vi "Dashboard Main.vi"() -> ()   [LabVIEW 2014]
uses:
  <vilib>/Rock Robotics/WPI/Camera/WPI_CameraSettings Read MJPG.ctl
  <vilib>/Rock Robotics/WPI/Camera/WPI_CameraImageSize.ctl
  Custom VIs/Examples/2015 Vision Example/Vision Support Code/Camera Types.ctl
  <vilib>/event_ctls.llb/eventvkey.ctl
  <vilib>/Rock Robotics/WPI/Dashboard/WPI_DashboardLogging Global.vi
  <vilib>/Rock Robotics/Network Tables/SD Write Number.vi
  <vilib>/Utility/config.llb/Write Key (String).vi
  <vilib>/Utility/config.llb/Write Key (I32).vi
  <vilib>/Utility/config.llb/NI_LVConfig.lvlib
  <vilib>/vision/NI_Vision_Development_Module.lvlib
panel:
  in  "Camera Address 2":string="USB 1"
  in  "Camera Settings 3":T1={"fps"=20, "compression"=30, "Image Size"=enum."320x240"}
  in  "TCP":refnum<k5>
  in  "Rec Mode":enum32{"Stop", "Record", "Playback"}(radio)
  in  "Vision":u16(ring) items=["Camera Off", "USB Camera SW", "USB Camera HW", "IP Camera"]
  out "Camera IP":string
  out "Image Message":string="Timeout in Camera Communications"
  in  "Dashboard Tab":T3(tab)
  in  "Camera Settings":T4={"Frame Rate"=30, "Compression"=30, "Size"=1} {"Frame Rate" scale=1.0..30.0; "Size" items=["640x480", "320x240", "160x120"]}
  out "MotorChart R":cluster{"Numeric":dbl, "Numeric":dbl}(graph)
  out "MotorChart L":T5(graph)
  out "MotorSliders R":cluster{"MotorSlide1":dbl, "MotorSlide2":dbl} {"MotorSlide2" scale=-1.0..1.0 scale format="%#_2e"; "MotorSlide1" scale=-1.0..1.0 scale format="%#_2e"}
  out "MotorSliders L":T6 {"MotorSlide4 2" scale=0.0..14.0 scale format="%#_2e"; "MotorSlide2" scale=-1.0..1.0 scale format="%#_2e"; "MotorSlide1" scale=-1.0..1.0 scale format="%#_2e"}
  out "JS1 Z":dbl(slide) scale=-1.0..1.0 scale format="%#_2e"
  out "JS1 Graph":cluster{"X":dbl, "Y":dbl}[](graph)
  out "JS1 Buttons":T7
  out "JS2 Z":dbl(slide) scale=-1.0..1.0 scale format="%#_2e"
  out "JS2 Graph":cluster{"X":dbl, "Y":dbl}[](graph)
  out "JS2 Buttons":T7
  out "Mode":T8(ring)=enum."Auto Disabled"
  in  "DB Camera Config":bool
  out "fps":dbl format="%#.1g"
  out "Mbps":dbl format="%#.1g"
  out "Mbps 2":bool
  in  "Carpet Color":T9(tab)
  in  "Red":T10={"Hue"={231.0, 14.0}, "Sat"={83.0, 255.0}, "Val"={52.5, 255.0}} {"Hue" scale=0.0..255.0 scale format="%#_3g"}
  in  "Blue":T10={"Hue"={119.0, 181.0}, "Sat"={33.0, 255.0}, "Val"={48.571428571428584, 255.0}} {"Hue" scale=0.0..255.0 scale format="%#_3g"}
  in  "Camera Type":T11=enum."MS HD3000 square"
  in  "Score Threshold":dbl=75.0
  in  "Annotate":bool=TRUE
  in  "Source":enum32{"Files", "Camera"}(tab)
  in  "Images":i32(listbox)
  in  "Folder Location":path=path "Sample Images/KicoffFilmingVision"
  in  "Camera Settings 2":T1={"fps"=20, "compression"=30, "Image Size"=enum."320x240"}
  in  "Camera Address":string="USB 1"
  in  "Show Mask?":bool
  in  "Limit Tests?":bool=TRUE
  in  "Show Carpet Mask":bool=TRUE
  in  "Aspect Fudge Factor":dbl=1.0
  in  "Tote Color":T10={"Hue"={23.67058792990901, 48.923317529462665}, "Sat"={66.78571428571429, 255.0}, "Val"={48.571428571428584, 255.0}} {"Hue" scale=0.0..255.0 scale format="%#_3g"}
  in  "Image Path":path=path "Sample Images/KicoffFilmingVision"
  in  "image files":string[](array[string])
  out "ms to process":u32
  out "Particles":i32
  out "Detected Totes":T12(array[cluster]) {"Normalized Rect"."Numeric 5" format="%#_2g"; "Normalized Rect"."Numeric 3" format="%#_2g"; "Normalized Rect"."Numeric 2" format="%#_2g"; "Normalized Rect"."Numeric" format="%#_2g"}
  out "Sorted Scores":T13(array[cluster]) {"Carpet" format="%#_3g"; "S" format="%#_3g"; "Trapezoid %" format="%#_3g"; "L" format="%#_3g"; "Area to CH" format="%#_3g"; "X" format="%#_3g"; "Y" format="%#_3g"}
  in  "Precision %":dbl(slide) scale=0.0..100.0
  in  "Test Slider":dbl(slide) scale=0.0..100.0 scale format="%#_3g"
  in  "On/Off":bool caption="Solenoid"
  in  "Test Name":u16(ring) items=["Select the test to run...", "Example Test", "-------------------------------", "List of tests is built in robot code.", "Replace with your own automated tests."]
  in  "Test Tree":string(tree)
  in  "Motor":cluster{"Value":dbl, "Enable":bool} {"Value" scale=-1.0..1.0 scale format="%#_3g"}
  out "Progress":T14 {"Test Progress" scale=0.0..100.0}
  in  "Rev/Fwd":cluster{"Forward":bool, "Reverse":bool}
  in  "Test Ring":u16(ring) items=["Monochrome", "Color"]
  in  "Listbox":i32(listbox)
  out "Tree":string(tree)
  out "Camera Image":T15(plugin-control)
  out "Boolean":bool
  # "Left"
  # "Front"
  # "Right"
  # "Battery"
  # "Aspect Ratio"
  # "Density Profile"
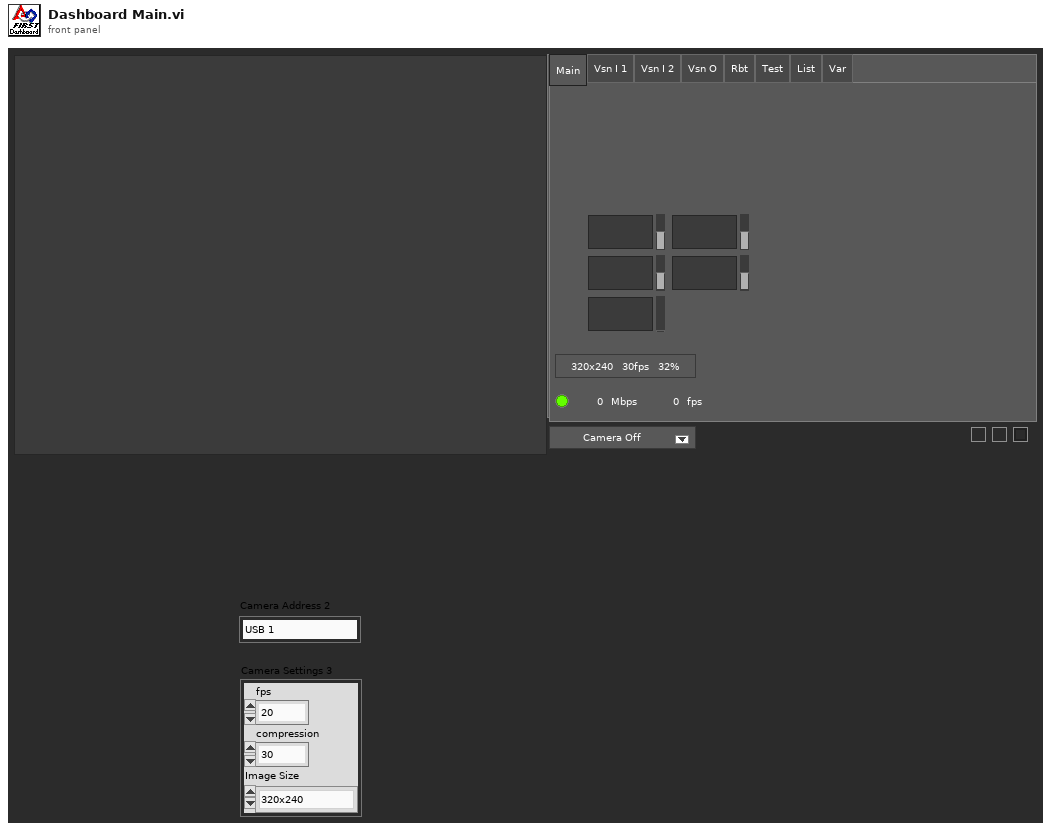
[diagram p1: front panel]
types:
  T1 = typedef "WPI_CameraSettings Read MJPG.ctl" = cluster{"fps":i32, "compression":i32, "Image Size":T2}
  T2 = typedef "WPI_CameraImageSize.ctl" = enum16{"640x480", "320x240", "160x120", "Custom"}
  T3 = enum32{"Main", "Vsn I 1", "Vsn I 2", "Vsn O", "Rbt", "Test", "List", "Var"}
  T4 = cluster{"Frame Rate":i32, "Compression":i32, "Size":u16}
  T5 = cluster{"Numeric":dbl, "Numeric":dbl, "Battery V":dbl}
  T6 = cluster{"MotorSlide1":dbl, "MotorSlide2":dbl, "MotorSlide4 2":dbl}
  T7 = cluster{bool, bool, bool, bool, bool, bool, bool, bool, bool, bool, bool, bool}
  T8 = enum8{"Tele-Op Disabled", "Tele-Op Enabled", "Auto Disabled", "Auto Enabled", "Test Disabled", "Test Enabled", "Disconnected", "No Code", "E-Stop"}
  T9 = enum32{"Red Carpet Color", "Blue Carpet Color", "None"}
  T10 = cluster{"Hue":cluster{dbl, dbl}, "Sat":cluster{dbl, dbl}, "Val":cluster{dbl, dbl}}
  T11 = typedef "Camera Types.ctl" = enum16{"206", "1011", "1013", "MS HD3000 square", "MS HD3000 640x480"}
  T12 = cluster{"Distance (ft)":dbl, "Center":cluster{dbl, dbl}, "Normalized Rect":cluster{"Numeric":dbl, "Numeric 2":dbl, "Numeric 3":dbl, "Numeric 5":dbl}}[]
  T13 = cluster{"Rectangle":cluster{"Numeric":dbl, "Numeric 2":dbl, "Numeric 3":dbl, "Numeric 5":dbl}, "Trapezoid %":dbl, "L":dbl, "S":dbl, "Area to CH":dbl, "X":dbl, "Y":dbl, "Carpet":dbl}[]
  T14 = cluster{"Test Progress":u8, "Test Progress Text":string}
  T15 = typedef "IMAQ Image.ctl" = refnum<image>
  T16 = typedef "Particle Parameters" = i32
  T17 = typedef "Image Type" = u32
  T18 = enum32{"Drive", "Basic", "Custom", "Test", "Checklist", "Variables"}
  T19 = cluster{"Camera Image":refnum<vi>, "Dashboard Tab":refnum<vi>, "Boolean":refnum<vi>, "Vision":refnum<vi>, "Rec Mode":refnum<vi>, "Test Slider":refnum<vi>, "On/Off ":refnum<vi>, "Test Ring":refnum<vi>, "Rev/Fwd":refnum<vi>, "Test Name":refnum<vi>, "Motor":refnum<vi>, "Progress":refnum<vi>, "CheckList":refnum<vi>, "Tree":refnum<vi>, "Test Tree":refnum<vi>}
  T20 = cluster{"Error Strings":string, "Disable Counts":cluster{u16, u16}, "Rail Faults":cluster{u16, u16, u16}, "Robot IP":string, "DB Mode":u8, "Event Info":cluster{"Name":string, "Type":u8, "Number":u16, "Replay":u8}, "Camera Addr":string}
  T21 = cluster{"Storage":cluster{"Disk Free":u64, "RAM Block":u32, "RAM free":u32}, "CPU Utilization":cluster{"CPU % ISR":sgl, "CPU % Time Crit":sgl, "CPU % Timed Str":sgl, "CPU % High":sgl, "CPU % Above":sgl, "CPU % Normal":sgl, "CPU % Low":sgl}, "CAN":cluster{"% Bus Utilization":sgl, "Bus Off Cnt":u32, "TX_FIFO Full Cnt":u32, "Receive Error Cnt":u8, "Transmit Error Cnt":u8}, "HID":cluster{"HID Outputs":u32, "Rumble Low":u16, "Rumble High":u16}[]}
  T22 = cluster{"Status bits":cluster{"Test Mode":bool, "Autonomous":bool, "Enabled":bool, "Code Start":bool, "Brownout":bool, "Reserved 2":bool, "Reserved 3":bool, "E-Stop":bool}, "Code Trace":cluster{"Disabled":bool, "TeleOp":bool, "Auto":bool, "Test":bool}, "Controller Type":enum16{"unknown", "cRIO", "roboRio"}, "Code?":enum16{"unknown", "noCode", "code"}, "Battery V":dbl}
  T23 = cluster{"Control Bits":cluster{"TestMode":bool, "Autonomous":bool, "Enabled":bool, "FMS Present":bool, bool, bool, bool, "E-Stop":bool}, "Team Station ":u8, "Countdown":sgl, "Joystick Values":cluster{"Axes":dbl[], "Buttons":bool[], "POVs":i16[]}[]}
  T24 = cluster{"Axes":dbl[], "Buttons":bool[], "POVs":i16[]}[]
  T25 = cluster{"Axes":dbl[], "Buttons":bool[], "POVs":i16[]}
  T26 = cluster{"Buttons[0]":bool, "Buttons[1]":bool, "Buttons[2]":bool, "Buttons[3]":bool, "Buttons[4]":bool, "Buttons[5]":bool, "Buttons[6]":bool, "Buttons[7]":bool, "Buttons[8]":bool, "Buttons[9]":bool, "Buttons[10]":bool, "Buttons[11]":bool}
  T27 = cluster{"Bounding box":cluster{"left":dbl, "top":dbl, "right":dbl, "bottom":dbl}, "Trapezoid":dbl, "Long Aspect":dbl, "Short Aspect":dbl, "Area to CH":dbl, "X Mask":dbl, "Y Mask":dbl, "Carpet":dbl}[]
  T28 = cluster{"Red":cluster{"Hue":cluster{dbl, dbl}, "Sat":cluster{dbl, dbl}, "Val":cluster{dbl, dbl}}, "Blue":cluster{"Hue":cluster{dbl, dbl}, "Sat":cluster{dbl, dbl}, "Val":cluster{dbl, dbl}}}
  T29 = cluster{cluster{"[0]":dbl, "[1]":dbl, "[2]":dbl, "[3]":dbl}, "Score":dbl, "Long Edge Score":dbl, "Short Edge Score":dbl, dbl, "X Score":dbl, "Y Score":dbl, "Carpet":dbl}[]
  T30 = cluster{"Found Totes[0]":cluster{"Distance (ft)":dbl, "Center":cluster{dbl, dbl}, "Normalized Rect":cluster{"Numeric":dbl, "Numeric 2":dbl, "Numeric 3":dbl, "Numeric 5":dbl}}, "Found Totes[1]":cluster{"Distance (ft)":dbl, "Center":cluster{dbl, dbl}, "Normalized Rect":cluster{"Numeric":dbl, "Numeric 2":dbl, "Numeric 3":dbl, "Numeric 5":dbl}}, "Found Totes[2]":cluster{"Distance (ft)":dbl, "Center":cluster{dbl, dbl}, "Normalized Rect":cluster{"Numeric":dbl, "Numeric 2":dbl, "Numeric 3":dbl, "Numeric 5":dbl}}, "Found Totes[3]":cluster{"Distance (ft)":dbl, "Center":cluster{dbl, dbl}, "Normalized Rect":cluster{"Numeric":dbl, "Numeric 2":dbl, "Numeric 3":dbl, "Numeric 5":dbl}}, "Found Totes[4]":cluster{"Distance (ft)":dbl, "Center":cluster{dbl, dbl}, "Normalized Rect":cluster{"Numeric":dbl, "Numeric 2":dbl, "Numeric 3":dbl, "Numeric 5":dbl}}, "Found Totes[5]":cluster{"Distance (ft)":dbl, "Center":cluster{dbl, dbl}, "Normalized Rect":cluster{"Numeric":dbl, "Numeric 2":dbl, "Numeric 3":dbl, "Numeric 5":dbl}}, "Found Totes[6]":cluster{"Distance (ft)":dbl, "Center":cluster{dbl, dbl}, "Normalized Rect":cluster{"Numeric":dbl, "Numeric 2":dbl, "Numeric 3":dbl, "Numeric 5":dbl}}, "Found Totes[7]":cluster{"Distance (ft)":dbl, "Center":cluster{dbl, dbl}, "Normalized Rect":cluster{"Numeric":dbl, "Numeric 2":dbl, "Numeric 3":dbl, "Numeric 5":dbl}}, "Found Totes[8]":cluster{"Distance (ft)":dbl, "Center":cluster{dbl, dbl}, "Normalized Rect":cluster{"Numeric":dbl, "Numeric 2":dbl, "Numeric 3":dbl, "Numeric 5":dbl}}}
  T31 = typedef "NI_LVConfig.lvlib/Config Data RefNum.ctl" = refnum<k1>
  T32 = cluster{"Operation":enum16{"Update", "Clear"}, "Color Box":u32}[]
  T33 = typedef "eventvkey.ctl" = enum16{"ASCII", "Enter", "Return", "Shift", "Ctrl", "Alt", "Cmd", "Opt", "Caps", "NumLock", "Clear", "Break", "Up", "Down", "Left", "Right", "Insert", "Delete", "Home", "End", "PageUp", "PageDown", "Escape", "Help", "Pause", "ScrollLock", "F1", "F2", "F3", "F4", "F5", "F6", "F7", "F8", "F9", "F10", "F11", "F12", "F13", "F14", "F15", "F16", "F17", "F18", "F19", "F20", "F21", "F22", "F23", "F24", "Play", "VolumeUp", "VolumeDown", "Mute", "Two Byte Char"}
  T34 = cluster{"Image Size":bool, "Image Type":bool, "Pixel Value":bool, "ROI Information":bool, "Zoom Factor":bool}
  T35 = enum8{"Enabled", "Disabled", "Disabled and Grayed Out"}
  T36 = cluster{"Operation":enum16{"Update", "Clear"}, "Color Box":u32}
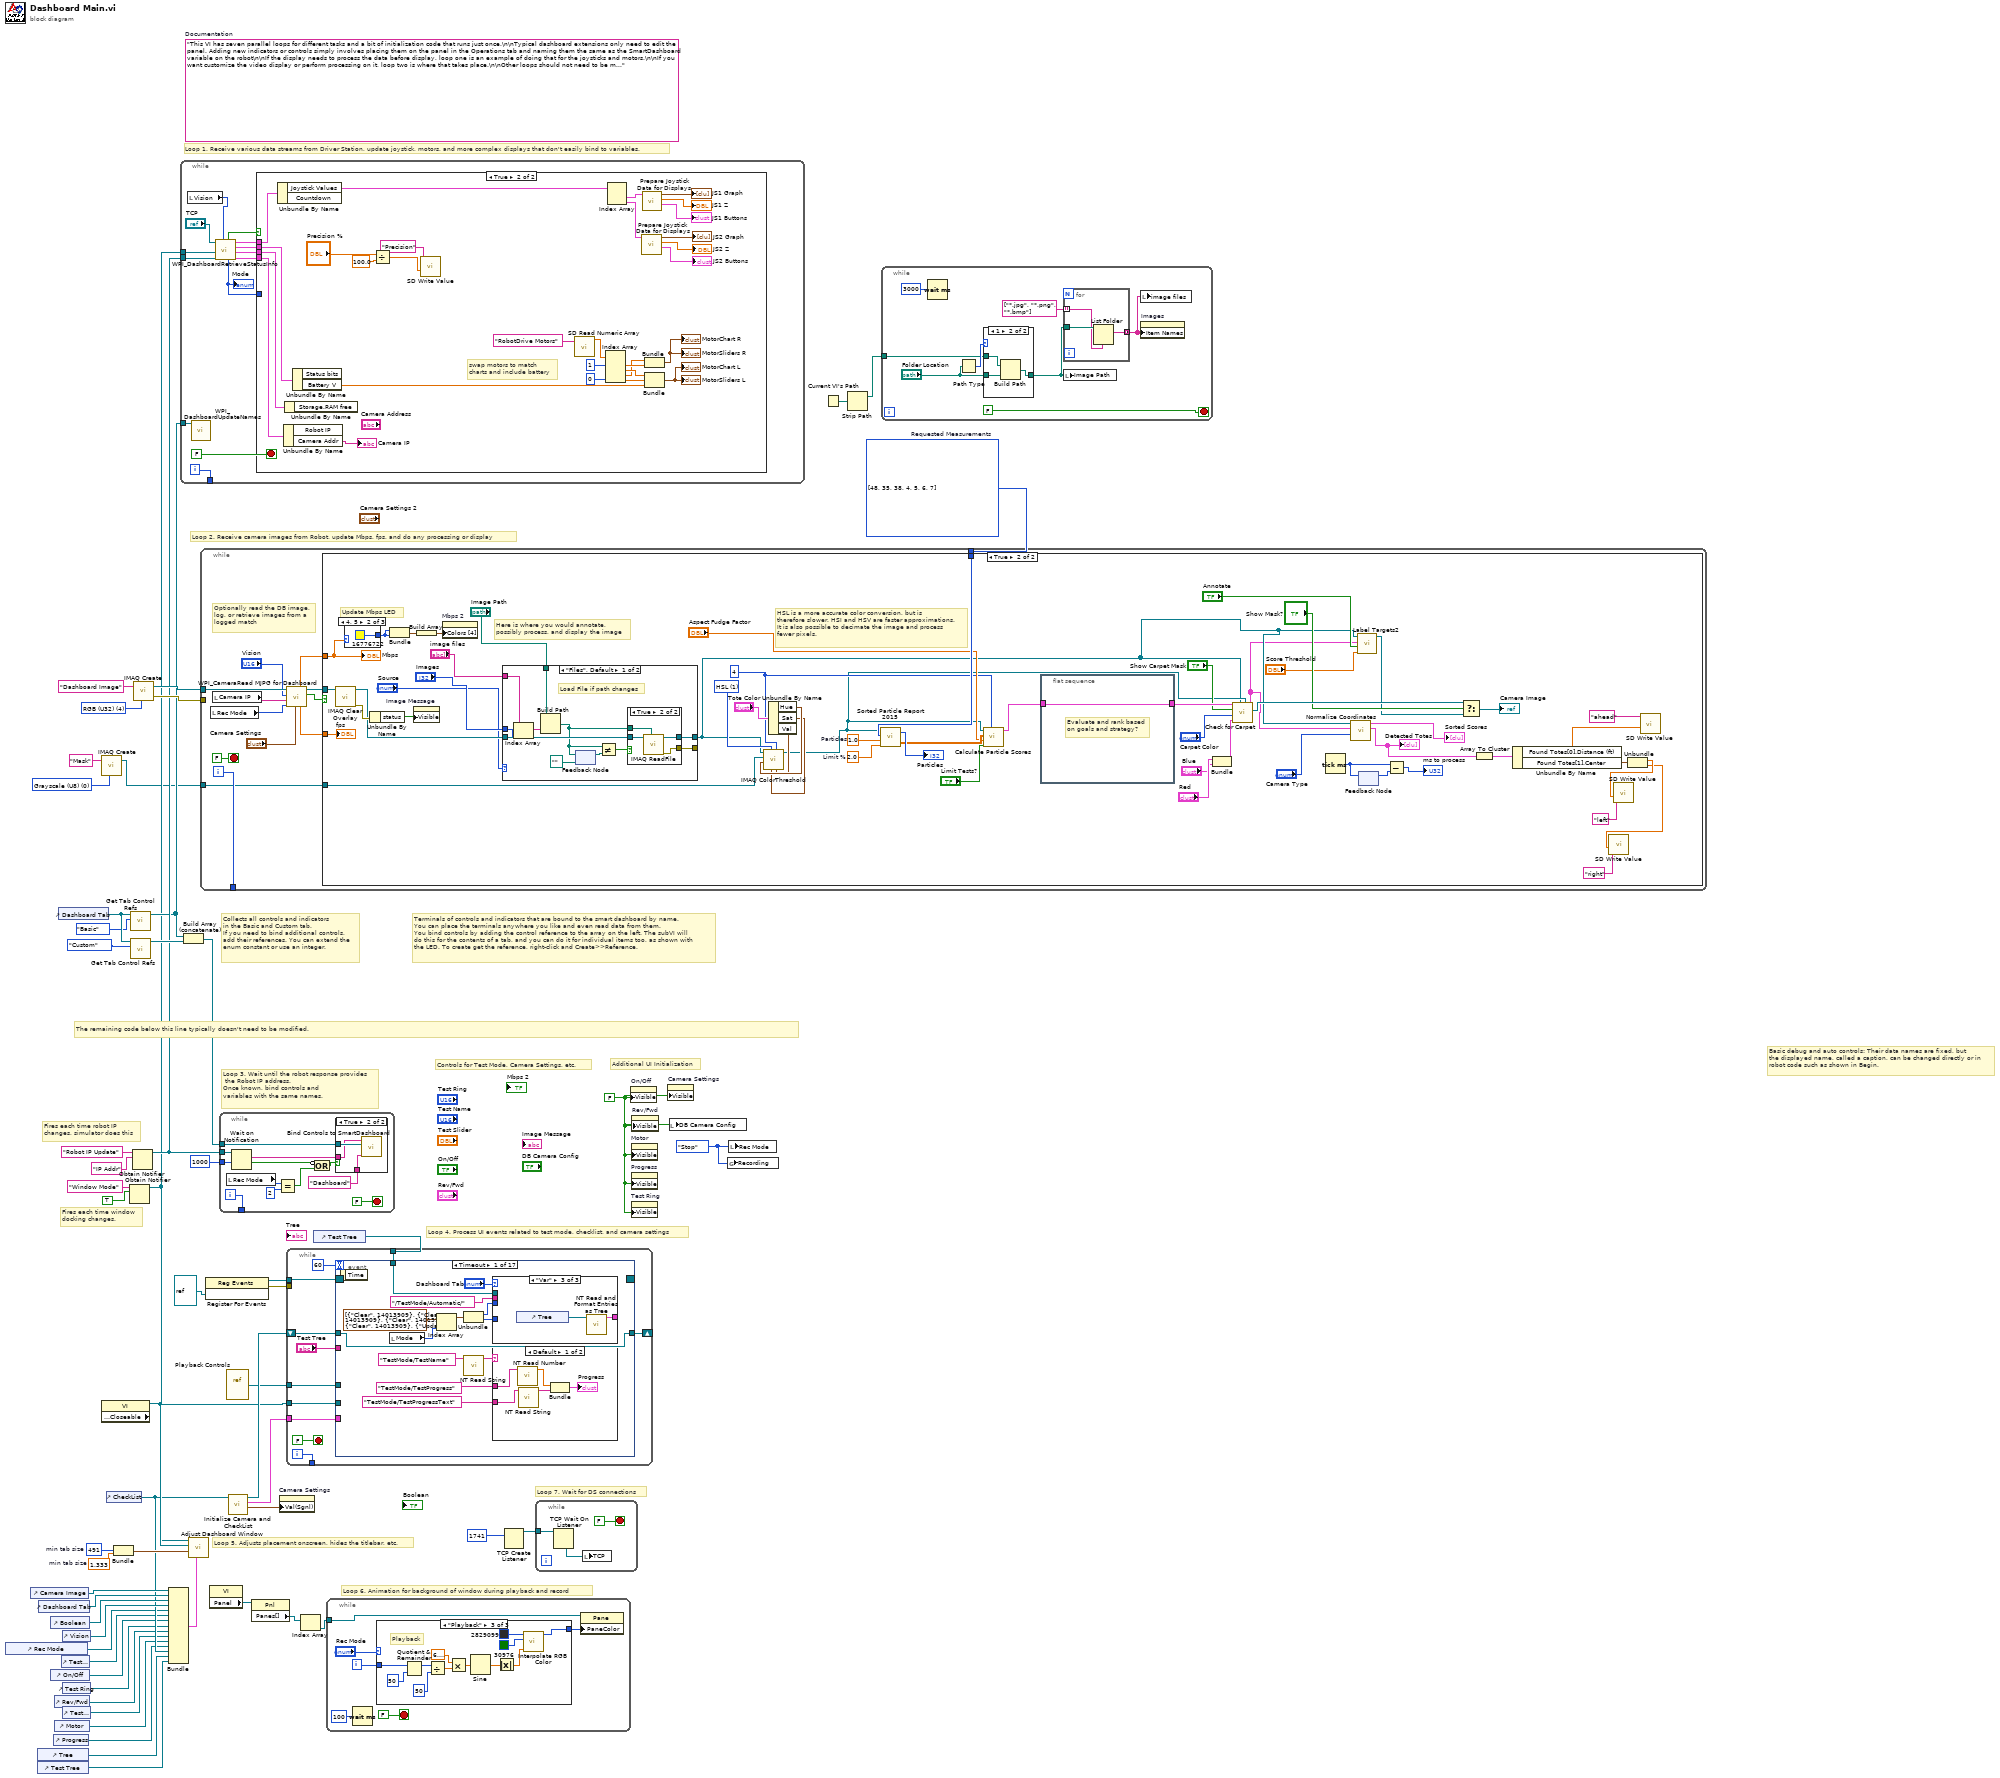
[diagram p0: block diagram]
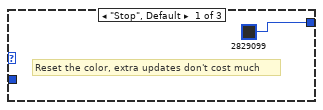
[diagram p4: hidden frame]
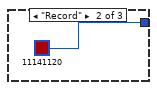
[diagram p5: hidden frame]
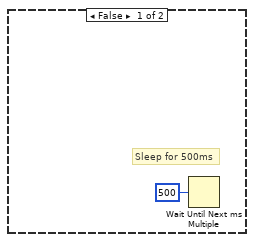
[diagram p7: hidden frame]
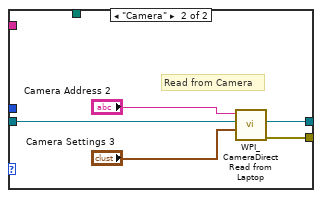
[diagram p9: hidden frame]
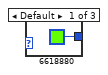
[diagram p10: hidden frame]
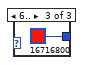
[diagram p11: hidden frame]
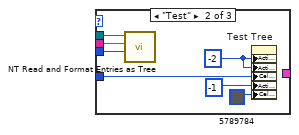
[diagram p13: hidden frame]
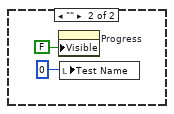
[diagram p14: hidden frame]
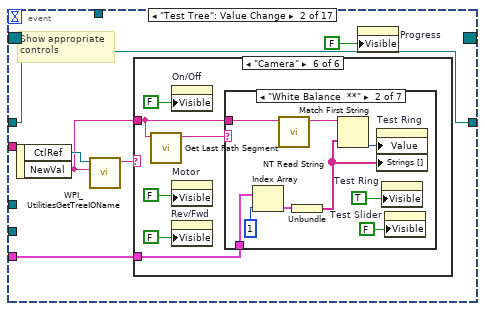
[diagram p15: hidden frame]
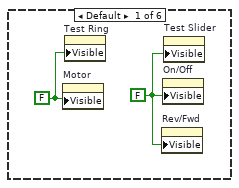
[diagram p16: hidden frame]
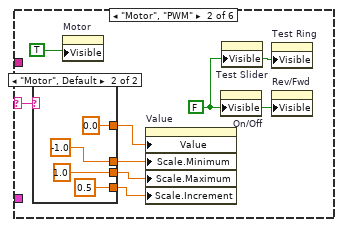
[diagram p17: hidden frame]
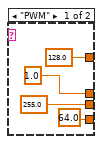
[diagram p18: hidden frame]
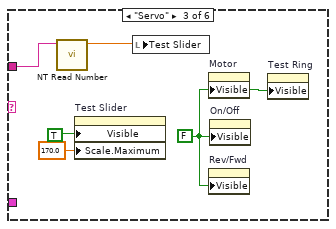
[diagram p19: hidden frame]
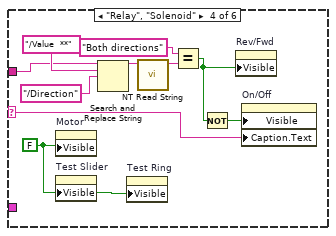
[diagram p20: hidden frame]
diagram:
  w1 = T16[] [48, 35, 38, 4, 5, 6, 7] items=["Center of Mass X", "Center of Mass Y", "First Pixel X", "First Pixel Y", "Bounding Rect Left", "Bounding Rect Top", "Bounding Rect Right", "Bounding Rect Bottom", "Max Feret Diameter Start X", "Max Feret Diameter Start Y", "Max Feret Diameter End X", "Max Feret Diameter End Y", "Max Horiz. Segment Length Left", "Max Horiz. Segment Length Right", "Max Horiz. Segment Length Row", "-", "Bounding Rect Width", "Bounding Rect Height", "Bounding Rect Diagonal", "Perimeter", "Convex Hull Perimeter", "Holes' Perimeter", "Max Feret Diameter", "Equivalent Ellipse Major Axis", "Equivalent Ellipse Minor Axis", "Equivalent Ellipse Minor Axis (Feret)", "Equivalent Rect Long Side", "Equivalent Rect Short Side", "Equivalent Rect Diagonal", "Equivalent Rect Short Side (Feret)", "Average Horiz. Segment Length", "Average Vert. Segment Length", "Hydraulic Radius", "Waddel Disk Diameter", "-", "Area", "Holes' Area", "Particle & Holes' Area", "Convex Hull Area", "Image Area", "-", "Number of Holes", "Number of Horiz. Segments", "Number of Vert. Segments", "-", "Orientation", "Max Feret Diameter Orientation", "-", "% Area/Image Area", "% Area/(Particle & Holes' Area)", "Ratio of Equivalent Ellipse Axes", "Ratio of Equivalent Rect Sides", "-", "Elongation Factor", "Compactness Factor", "Heywood Circularity Factor", "Type Factor", "-", "Sum X", "Sum Y", "Sum XX", "Sum XY", "Sum YY", "Sum XXX", "Sum XXY", "Sum XYY", "Sum YYY", "-", "Moment of Inertia XX", "Moment of Inertia XY", "Moment of Inertia YY", "Moment of Inertia XXX", "Moment of Inertia XXY", "Moment of Inertia XYY", "Moment of Inertia YYY", "Norm. Moment of Inertia XX", "Norm. Moment of Inertia XY", "Norm. Moment of Inertia YY", "Norm. Moment of Inertia XXX", "Norm. Moment of Inertia XXY", "Norm. Moment of Inertia XYY", "Norm. Moment of Inertia YYY", "Hu Moment 1", "Hu Moment 2", "Hu Moment 3", "Hu Moment 4", "Hu Moment 5", "Hu Moment 6", "Hu Moment 7"]  # Requested Measurements
  w4 = T17 0 items=["Grayscale (U8)", "Grayscale (I16)", "Grayscale (SGL)", "Complex (CSG)", "RGB (U32)", "HSL (U32)", "RGB (U64)", "Grayscale (U16)"] ("Image Type")
  w30 = 491  # min tab size
  w29 = 1.333  # min tab size
  w38 = enum32{"Stop", "Record", "Playback"}."Stop" ("Rec Mode")
  w12 = FALSE ("Visible")
  (unwired) "This VI has seven parallel loops for different tasks and a bit of initialization code that runs just once.\n\nTypical dashboard extensions only need to edit the panel. Adding new indicators or controls simply involves placing them on the panel in the Operations tab and naming them the same as the SmartDashboard variable on the robot\n\nIf the display needs to process the data before display, loop one is an example of doing that for the joysticks and motors.\n\nIf you want customize the video display or perform processing on it, loop two is where that takes place.\n\nOther loops should not need to be modified. They are pretty standard, and document the task they perform."  # Documentation
  w58 = T17 4 items=["Grayscale (U8)", "Grayscale (I16)", "Grayscale (SGL)", "Complex (CSG)", "RGB (U32)", "HSL (U32)", "RGB (U64)"] ("Image Type")
  # "Loop 7. Wait for DS connections"
  # "Basic debug and auto controls: Their data names are fixed, but\nthe displayed name, called a caption, can be changed directly or in\nrobot code such as shown in Begin."
  # "Controls for Test Mode, Camera Settings, etc."
  # "Additional UI Initialization"
  # "Loop 6. Animation for background of window during playback and record"
  # "Fires each time robot IP\nchanges, simulator does this"
  # "Fires each time window\ndocking changes."
  # "Collects all controls and indicators\nin the Basic and Custom tab.\nIf you need to bind additional controls,\nadd their references. You can extend the\nenum constant or use an integer."
  # "The remaining code below this line typically doesn't need to be modified."
  # "Loop 4. Process UI events related to test mode, checklist, and camera settings"
  # "Terminals of controls and indicators that are bound to the smart dashboard by name.\nYou can place the terminals anywhere you like and even read data from them.\nYou bind controls by adding the control reference to the array on the left. The subVI will\ndo this for the contents of a tab, and you can do it for individual items too, as shown with\nthe LED. To create get the reference, right-click and Create>>Reference."
  # "Loop 3. Wait until the robot response provides\n the Robot IP address.\nOnce known, bind controls and\nvariables with the same names."
  # "Loop 5. Adjusts placement onscreen, hides the titlebar, etc."
  # "Loop 1. Receive various data streams from Driver Station, update joystick, motors, and more complex displays that don't easily bind to variables."
  # "Loop 2. Receive camera images from Robot, update Mbps, fps, and do any processing or display"
  n1 = control-ref of="Rec Mode"() -> (w18:refnum<vi>)
  n2 = control-ref of="Camera Image"() -> (w33:refnum<vi>)
  n3 = control-ref of="Tree"() -> (w22:refnum<vi>)
  n4 = control-ref of="Test Tree"() -> (w21:refnum<vi>)
  n5 = control-ref of="Dashboard Tab"() -> (w32:refnum<vi>)
  n6 = control-ref of="Boolean"() -> (w27:refnum<vi>)
  n7 = control-ref of="On/Off"() -> (w16:refnum<vi>)
  n8 = control-ref of="Progress"() -> (w13:refnum<vi>)
  n9 = control-ref of="Rev/Fwd"() -> (w14:refnum<vi>)
  n10 = control-ref of="Motor"() -> (w19:refnum<vi>)
  n11 = control-ref of="Dashboard Tab"() -> (w36:refnum<vi>)
  n12 = control-ref of="Test Slider"() -> (w17:refnum<vi>)
  n13 = control-ref of="Vision"() -> (w31:refnum<vi>)
  n14 = control-ref of="Test Ring"() -> (w15:refnum<vi>)
  n15 = control-ref of="Test Name"() -> (w20:refnum<vi>)
  n16 = call "IMAQ Create"("Image Name"="Mask", "Image Type"=w4) -> ("New Image"=w2:T15)  [unwired: 2 in, 2 out]
  n17 = property class="VI" props=["Front Panel.Closeable"]() -> (reference out=w37:refnum<vi>)  [unwired: 2 in, 2 out]
  n18 = control-ref of="CheckList"() -> (w23:refnum<vi>)
  n19 = Bundle("min tab size"=w30, "min tab size"=w29) -> (w28:cluster{"min tab size":i32, "min tab size":dbl})  [unwired: 1 in]
  n20 = Obtain Notifier(name (unnamed)="Window Mode", notification data type=TRUE) -> (notifier out=w9:refnum<notifier>)  [unwired: 2 in, 2 out]
  n21 = call <vilib>:"Get Tab Control Refs.vi"("Page Index"=T18."Basic" ("Dashboard Tab"), "TabControl in"=w36) -> ("ControlsOnPage"=w10:refnum<vi>[])  [unwired: 9 in]
  n22 = call <vilib>:"Get Tab Control Refs.vi"("Page Index"=T18."Custom" ("Dashboard Tab"), "TabControl in"=w36) -> ("ControlsOnPage"=w35:refnum<vi>[])  [unwired: 9 in]
  n23 = Obtain Notifier(name (unnamed)="Robot IP Update", notification data type="IP Addr" ("name (unnamed)")) -> (notifier out=w11:refnum<notifier>)  [unwired: 2 in, 2 out]
  n24 = call "IMAQ Create"("Image Name"="Dashboard Image", "Image Type"=w58) -> ("New Image"=w56:T15, "error out"=w55:errorcluster)  [unwired: 2 in, 1 out]
  n25 = Bundle("Camera Image"=w33, "Dashboard Tab"=w32, "Boolean"=w27, "Vision"=w31, "Rec Mode"=w18, "Test Slider"=w17, "On/Off"=w16, "Test Ring"=w15, "Rev/Fwd"=w14, "Test Name"=w20, "Motor"=w19, "Progress"=w13, "CheckList"=w23, "Tree"=w22, "Test Tree"=w21) -> (w24:T19)  [unwired: 1 in]
  n26 = while {
    tunnel: [w70] -> _
    tunnel: w11 -> [w64]
    tunnel: w10 -> [w63]
    tunnel: w9 -> [w59]
    i -> [w70]
    stop <- FALSE stop-if-true
    n27 = local read "Vision"() -> (w61:u16)
    n28 = call <vilib>:"WPI_DashboardUpdateNames.vi"("Controls on Tab"=w63) -> ()  [unwired: 11 in]
    n29 = call <vilib>:"WPI_DashboardRetrieveStatusInfo.vi"("Vision"=w61, "Binding Refnum"=w64, "Window Mode Notifier"=w59, "TCP Cnx"="TCP") -> ("Power and Errors"=w65:T20, "Robot Metrics"=w68:T21, "Status Info"=w69:T22, "Control Info"=w66:T23, "Robot Mode"=w62:T8, "Process?"=w67:bool)  [unwired: 2 in]
    "Mode" <- w62
    n30 = case shown="True" w67 {
      tunnel: w69 -> [_ w100]
      tunnel: w68 -> [_ w99]
      tunnel: w66 -> [_ w98]
      tunnel: w65 -> [_ w97]
      tunnel: w62 -> [_ _]
      frame False {
      }
      frame True {
        # "swap motors to match\ncharts and include battery"
        n31 = Unbundle By Name(w98) -> ("Joystick Values"=w85:T24)  [unwired: 1 out]
        n32 = Unbundle By Name(w97) -> ("Camera Addr"=→"Camera IP":string)  [unwired: 1 out]
        n33 = Unbundle By Name(w99) -> ()  [unwired: 1 out]
        n34 = Unbundle By Name(w100) -> ("Battery V"=w86:dbl)  [unwired: 1 out]
        n35 = Divide(x="Precision %", y=100.0) -> (x/y=w73:dbl)
        n36 = call-poly <vilib>:"SD Write Value.vi"("Numeric"=w73, "Name"="Precision") -> ()  [unwired: 8 in, 2 out]
        n37 = call <vilib>:"SD Read Numeric Array.vi"("Name"="RobotDrive Motors") -> ("Numeric Array"=w88:dbl[])  [unwired: 8 in, 2 out]
        n38 = Index Array(array=w88, index #1=1, index #4=0) -> (element #1=w92:dbl, element #2=w93:dbl, element #3=w91:dbl, element #4=w96:dbl)  [unwired: 2 in]
        n39 = Index Array(array=w85) -> (element #1=w84:T25, element #2=w79:T25)  [unwired: 2 in]
        n40 = call "Prepare Joystick Data for Displays.vi"("Joystick Values"=w79) -> ("Buttons"=→"JS2 Buttons":T26, "Z Axis"=→"JS2 Z":dbl, "Cartesian Data"=→"JS2 Graph":cluster{"X axis":dbl, "X axis":dbl}[])  [unwired: 8 in]
        n41 = call "Prepare Joystick Data for Displays.vi"("Joystick Values"=w84) -> ("Buttons"=→"JS1 Buttons":T26, "Z Axis"=→"JS1 Z":dbl, "Cartesian Data"=→"JS1 Graph":cluster{"X axis":dbl, "X axis":dbl}[])  [unwired: 8 in]
        n42 = Bundle("Numeric"=w91, "Numeric"=w92) -> (→"MotorChart R" →"MotorSliders R":cluster{"Numeric":dbl, "Numeric":dbl})  [unwired: 1 in]
        n43 = Bundle("Numeric"=w93, "Numeric"=w96, "Battery V"=w86) -> (→"MotorChart L" →"MotorSliders L":T5)  [unwired: 1 in]
      }
    }
  }
  n44 = Build Array (concatenate)(w10, w35) -> (w34:refnum<vi>[])
  n45 = call "Adjust Dashboard Window.vi"("Sizing Refnums"=w24, "Size Constraints"=w28, "VI"=w37, "Notifier in"=w9) -> ()  [unwired: 8 in]
  n46 = while {
    tunnel: w56 -> [w111]
    tunnel: w55 -> [_]
    tunnel: [w112] -> _
    tunnel: w2 -> [w102]
    tunnel: w1 -> [w101]
    i -> [w112]
    stop <- FALSE stop-if-true
    # "Optionally read the DB image,\nlog, or retrieve images from a\nlogged match"
    n47 = local read "Rec Mode"() -> (w105:enum32{"Stop", "Record", "Playback"})
    n48 = local read "Camera IP"() -> (w103:string)
    n49 = call <vilib>:"WPI_CameraRead MJPG for Dashboard.vi"("Camera Settings"="Camera Settings", "Rec Mode"=w105, "Camera IP"=w103, "Camera Mode"="Vision", "Refnum in"=w111) -> ("Active"=w109:bool, "Refnum out"=w110:T15, "FPS"=w108:dbl, "Bandwidth (Mbps)"=w107:dbl)  [unwired: 3 in]
    n50 = case shown="True" w109 {
      tunnel: w110 -> [_ w166]
      tunnel: w107 -> [_ w165]
      tunnel: w108 -> [_ w164]
      tunnel: w102 -> [_ w158]
      tunnel: w101 -> [_ w150]
      frame False {
        # "Sleep for 500ms"
        n51 = Wait Until Next ms Multiple(millisecond multiple=u32 500) -> ()  [unwired: 1 out]
      }
      frame True {
        w151 = 2.0  # Limit %
        w152 = 1.0  # Particles
        w145 = 4 ("Replace Value")
        w153 = u16 1 items=["RGB", "HSL", "HSV", "HSI"] ("Color Mode")
        # "HSL is a more accurate color conversion, but is\ntherefore slower. HSI and HSV are faster approximations.\nIt is also possible to decimate the image and process\nfewer pixels."
        # "Here is where you would annotate,\npossibly process, and display the image"
        # "Update Mbps LED"
        n52 = call "IMAQ Clear Overlay"("Image"=w166) -> ("error out"=w170:errorcluster, "Image Out"=w161:T15)  [unwired: 2 in, 7 out]
        n53 = case shown="4, 5" w165 {
          tunnel: [u32 6618880 ("Color Box") u32 16776722 ("Color Box") u32 16716800 ("Color Box")] -> w167
          frame Default {
          }
          frame 4, 5 {
          }
          frame 6.. {
          }
        }
        n54 = Unbundle By Name(w170) -> ("status"=w171:bool)
        n55 = Bundle("Color Box"=w167, "Color Box"=w167) -> (w169:cluster{"Color Box":u32, "Color Box":u32})  [unwired: 1 out]
        n56 = property on="Image Message" class="Str"("Visible"=w171) -> ()  [unwired: 2 in, 2 out]
        n57 = Build Array(w169) -> (w168:cluster{"Color Box":u32, "Color Box":u32}[])
        n58 = property on="Mbps 2" class="Bool (strict)"("Colors [4]"=w168) -> ()  [unwired: 2 in, 2 out]
        n59 = case shown="\"Files\", Default" "Source" {
          tunnel: [w182 w193] -> _
          tunnel: [w183 w192] -> w127
          tunnel: w161 -> [w181 w191]
          tunnel: "image files" -> [w173 _]
          tunnel: "Images" -> [w180 _]
          tunnel: "Image Path" -> [w178 _]
          frame "Files", Default {
            # "Load File if path changes"
            n60 = Index Array(array=w173, index=w180) -> (element=w179:string)
            n61 = Build Path(base path=w178, name or relative path=w179) -> (appended path=w174:path)
            n62 = feedback-in #1(w174) -> ()
            n63 = feedback #1(path "" ("appended path")) -> (w176:path)
            n64 = Not Equal?(x=w174, y=w176) -> (x != y?=w177:bool)
            n65 = case shown="True" w177 {
              tunnel: [w184 w188] -> w183
              tunnel: [_ w187] -> w182
              tunnel: w181 -> [w184 w186]
              tunnel: w174 -> [_ w185]
              frame False {
              }
              frame True {
                n66 = call "IMAQ ReadFile"("File Path"=w185, "Image"=w186) -> ("error out"=w187:errorcluster, "Image Out"=w188:T15)  [unwired: 5 in, 3 out]
              }
            }
          }
          frame "Camera" {
            # "Read from Camera"
            n67 = call <vilib>:"WPI_CameraDirect Read from Laptop.vi"("Camera Settings"="Camera Settings 3", "Image"=w191, "address"="Camera Address 2") -> ("error out"=w193:errorcluster, "Image Out"=w192:T15)  [unwired: 7 in]
          }
        }
        n68 = Unbundle By Name("Tote Color") -> ("Hue"=w156:cluster{dbl, dbl}, "Sat"=w155:cluster{dbl, dbl}, "Val"=w154:cluster{dbl, dbl})
        n69 = call "IMAQ ColorThreshold"("Blue or Luma or Val or Inten Range"=w154, "Replace Value"=w145, "Green or Sat Range"=w155, "Color Mode"=w153, "Red or Hue Range"=w156, "Image Dst"=w158, "Image Src"=w127) -> ("Image Dst Out"=w137:T15)  [unwired: 3 in, 1 out]
        n70 = call "Sorted Particle Report 2015.vi"("Min Area Size %"=w151, "Particle Count Limit"=w152, "Pixel Measurements"=w150, "Image in"=w137) -> ("Sorted Data"=w148:dbl[][], "Particles"=→"Particles":i32)
        n71 = call "Calculate Particle Scores.vi"("Pixel Value"=w145, "Limit Tests?"="Limit Tests?", "Aspect Fudge Factor"="Aspect Fudge Factor", "Sorted Data"=w148, "Image in"=w137) -> ("Scores"=w144:T27)  [unwired: 6 in]
        n72 = flat-sequence {
          tunnel: w144 -> [w172]
          tunnel: [w172] -> w143
          frame #0 {
            # "Evaluate and rank based\non goals and strategy?"
          }
        }
        n73 = Bundle("Red"="Red", "Blue"="Blue") -> (w138:T28)  [unwired: 1 in]
        n74 = call "Check for Carpet.vi"("Original Mask"=w137, "Original Color"=w127, "Carpet Colors"=w138, "Carpet Selector"="Carpet Color", "Combine Carpet Mask"="Show Carpet Mask", "Initial Scores"=w143) -> ("Updated Mask"=w136:T15, "Updated Scores"=w126:T29)  [unwired: 4 in]
        n75 = Tick Count (ms)() -> (millisecond timer value=w133:u32)
        n76 = call "Normalize Coordinates.vi"("Camera Type"="Camera Type", "Targets"=w126, "Image in"=w127) -> ("Found Totes"=w123:T12, "Sorted Scores"=→"Sorted Scores":T13)  [unwired: 7 in]
        "Detected Totes" <- w123
        n77 = call "Label Targets2.vi"("Score Threshold"="Score Threshold", "Annotate"="Annotate", "Targets"=w126, "Image in"=w127) -> ("Image out"=w130:T15)  [unwired: 7 in]
        n78 = feedback #2() -> (w134:u32)  [unwired: 1 in]
        n79 = feedback-in #2(w133) -> ()
        n80 = Subtract(x=w133, y=w134) -> (x-y=→"ms to process":u32)
        n81 = Select(t=w136, s="Show Mask?", f=w130) -> (s? t:f=→"Camera Image":T15)
        n82 = Array To Cluster(array=w123) -> (cluster=w122:T30)
        n83 = Unbundle By Name(w122) -> ("Found Totes[0].Distance (ft)"=w120:dbl, "Found Totes[1].Center"=w121:cluster{dbl, dbl})
        n84 = Unbundle(w121) -> (w119:dbl, w118:dbl)
        n85 = call-poly <vilib>:"SD Write Value.vi"("Numeric"=w118, "Name"="right") -> ()  [unwired: 8 in, 2 out]
        n86 = call-poly <vilib>:"SD Write Value.vi"("Numeric"=w119, "Name"="left") -> ()  [unwired: 8 in, 2 out]
        n87 = call-poly <vilib>:"SD Write Value.vi"("Numeric"=w120, "Name"="ahead") -> ()  [unwired: 8 in, 2 out]
        "Mbps" <- w165
        "fps" <- w164
      }
    }
  }
  n88 = register-events(refnum<vi> refnum) -> (reference out=w42:refnum<event-registration>, error out=w41:errorcluster)  [unwired: 2 in]
  n89 = property class="VI"() -> ("Panel"=w45:refnum<vi>)  [unwired: 2 in, 2 out]
  n90 = while {
    tunnel: w34 -> [w208]
    tunnel: w11 -> [w206]
    tunnel: [w204] -> _
    tunnel: u32 1000 ("milliseconds to wait") -> [w203]
    i -> [w204]
    stop <- FALSE stop-if-true
    n91 = local read "Rec Mode"() -> (w199:enum32{"Stop", "Record", "Playback"})
    n92 = Wait on Notification(notifier=w206, timeout in ms (-1)=w203) -> (notification=w205:string, timed out?=w201:bool)  [unwired: 2 in, 2 out]
    n93 = Equal?(x=w199, y=u16 2 ("Rec Mode")) -> (x = y?=w200:bool)
    n94 = Compound Arithmetic op=OR(invert w201, w200) -> (w202:bool)
    n95 = case shown="True" w202 {
      tunnel: w208 -> [_ w211]
      tunnel: w205 -> [_ w210]
      tunnel: "Dashboard" -> [_ w209]
      frame False {
      }
      frame True {
        n96 = call <vilib>:"Bind Controls to SmartDashboard.vi"("Client Name"=w209, "Bound Control Refs"=w211, "Server IP Address"=w210) -> ()  [unwired: 9 in]
      }
    }
  }
  n97 = vi-ref "Playback Controls.vi"() -> (w43:refnum<vi>)
  n98 = call "Initialize Camera and CheckList.vi"("ListBox in"=w23) -> ("Cluster"=w49:cluster{"value":i32, "value":i32, "index":i32}, "Array"=w50:cluster{string[]}[], "File Refnum"=w48:T31)  [unwired: 8 in]
  n99 = property class="Pnl"(reference=w45) -> ("Panes[]"=w46:refnum<vi>[])  [unwired: 1 in, 2 out]
  n100 = property on="Camera Settings" class="Clust (strict)"("Val(Sgnl)"=w49) -> ()  [unwired: 2 in, 2 out]
  n101 = Index Array(array=w46) -> (element=w44:refnum<vi>)  [unwired: 1 in]
  n102 = control-ref of="Test Tree"() -> (w47:refnum<vi>)
  n103 = while {
    tunnel: w50 -> [w219]
    shift-right: [w218] -> _
    shift-left: w48 -> [w217]
    tunnel: [w216] -> _
    tunnel: w47 -> [w215]
    tunnel: w43 -> [w214]
    tunnel: w42 -> [w213]
    tunnel: w41 -> [_]
    tunnel: w37 -> [w212]
    i -> [w216]
    stop <- FALSE stop-if-true
    n104 = event shown="[0] Timeout" {
      selector: w213 -> [_ _ _ _ _ _ _ _ _ _ _ _ _ _ _ _ _]
      dyn-events: [_ _ _ _ _ _ _ _ _ _ _ _ _ w457 _ _ _] -> _
      timeout: u32 60 ("milliseconds to wait") -> [_ _ _ _ _ _ _ _ _ _ _ _ _ _ _ _ _]
      tunnel: w215 -> [w231 _ _ _ _ _ _ _ _ _ _ _ _ _ _ _ _]
      tunnel: "Test Tree" -> [_ _ _ _ _ _ _ _ w426 w434 w436 w440 w448 _ _ _ _]
      tunnel: w219 -> [_ w253 _ _ _ _ w390 w420 _ _ _ _ _ _ _ _ _]
      tunnel: [w227 w252 w351 w356 w364 w376 w389 w413 w425 w432 w435 w439 w447 w459 w473 w474 w484] -> w218
      tunnel: w217 -> [w227 w252 w351 w356 w364 w376 w388 w413 w425 w432 w435 w439 w447 w459 w473 w474 w484]
      tunnel: w214 -> [_ _ _ _ _ _ _ _ _ _ _ _ _ w460 _ w477 _]
      tunnel: w212 -> [_ _ _ _ _ _ _ _ _ _ _ _ _ w455 _ _ _]
      event Timeout {
        n105 = event-data() -> ()  [unwired: 1 in, 1 out]
        n106 = local read "Mode"() -> (w230:T8)
        n107 = Index Array(array=T32 [{"Operation"=enum."Clear", "Color Box"=14013909}, {"Operation"=enum."Clear", "Color Box"=14013909}, {"Operation"=enum."Clear", "Color Box"=14013909}, {"Operation"=enum."Clear", "Color Box"=14013909}, {"Operation"=enum."Update", "Color Box"=14013909}, {"Operation"=enum."Update", "Color Box"=16777215}, {"Operation"=enum."Clear", "Color Box"=14013909}, {"Operation"=enum."Clear", "Color Box"=14013909}, {"Operation"=enum."Clear", "Color Box"=14013909}], index=w230) -> (element=w225:T36)
        n108 = Unbundle(w225) -> ("Operation"=w224:enum16{"Update", "Clear"}, "Color Box"=w223:u32)
        n109 = call <vilib>:"NT Read String.vi"("Name"="TestMode/TestName") -> ("String"=w234:string)  [unwired: 9 in, 1 out]
        n110 = case shown="\"Var\"" "Dashboard Tab" {
          tunnel: w231 -> [_ w242 _]
          tunnel: "/TestMode/Automatic/" ("Name Pattern") -> [_ w241 _]
          tunnel: w224 -> [_ w240 _]
          tunnel: [_ _ w244] -> _
          tunnel: w223 -> [_ w236 _]
          frame "Rbt", Default {
          }
          frame "Test" {
            w239 = -2 ("Active Item:Row Number")
            n111 = call <vilib>:"NT Read and Format Entries as Tree.vi"("Operation"=w240, "Name Pattern"=w241, "Tree Refnum"=w242) -> ()  [unwired: 7 in, 2 out]
            n112 = property on="Test Tree" class="Tree (strict)"("Active Item Row Number"=w239, "ActiveColNum"=w239, "CellBG"=w236, "Active Item Row Number"=-1 ("Active Item:Row Number"), "CellBG"=u32 5789784 ("Color Box")) -> ()  [unwired: 2 in, 2 out]
          }
          frame "Var" {
            n113 = control-ref of="Tree"() -> (w243:refnum<vi>)
            n114 = call <vilib>:"NT Read and Format Entries as Tree.vi"("Tree Refnum"=w243) -> ("Formatted Strings"=w244:cluster{"Name":string, "Value":string}[])  [unwired: 9 in, 1 out]
          }
        }
        n115 = case shown="Default" w234 {
          tunnel: "TestMode/TestProgress" ("Name") -> [w246 _]
          tunnel: "TestMode/TestProgressText" ("Name") -> [w245 _]
          frame Default {
            n116 = call <vilib>:"NT Read Number.vi"("Name"=w246) -> ("Numeric"=w247:dbl)  [unwired: 9 in, 1 out]
            n117 = call <vilib>:"NT Read String.vi"("Name"=w245) -> ("String"=w248:string)  [unwired: 9 in, 1 out]
            n118 = Bundle("Numeric"=w247, "String"=w248) -> (→"Progress":cluster{"Numeric":dbl, "String":string})  [unwired: 1 in]
          }
          frame "" {
            n119 = property on="Progress" class="Clust (strict)"("Visible"=FALSE) -> ()  [unwired: 2 in, 2 out]
            n120 = local write "Test Name"(u16 0) -> ()
          }
        }
      }
      event "Test Tree": Value Change {
        # "Show appropriate\ncontrols"
        n121 = event-data() -> ("CtlRef"=w256:refnum<vi>, "NewVal"=w254:string)  [unwired: 1 in]
        n122 = call <vilib>:"WPI_UtilitiesGetTreeIOName.vi"("NewVal"=w254, "TreeControl in"=w256) -> ("I/O Name"=w257:string)  [unwired: 9 in]
        n123 = case shown="\"Camera\"" w257 {
          selector: w257 -> [_ w264 _ w282 w291 _]
          tunnel: w254 -> [_ _ w279 w281 _ w298]
          tunnel: w253 -> [_ _ _ _ _ w297]
          frame Default {
            w259 = FALSE ("Visible")
            w258 = FALSE ("Visible")
            n124 = property on="Motor" class="Clust (strict)"("Visible"=w258) -> ()  [unwired: 2 in, 2 out]
            n125 = property on="Test Ring" class="Ring (strict)"("Visible"=w258) -> ()  [unwired: 2 in, 2 out]
            n126 = property on="Rev/Fwd" class="Clust (strict)"("Visible"=w259) -> ()  [unwired: 2 in, 2 out]
            n127 = property on="On/Off" class="Bool (strict)"("Visible"=w259) -> ()  [unwired: 2 in, 2 out]
            n128 = property on="Test Slider" class="Slide (strict)"("Visible"=w259) -> ()  [unwired: 2 in, 2 out]
          }
          frame "Motor", "PWM" {
            w265 = FALSE ("Visible")
            n129 = case shown="\"Motor\", Default" w264 {
              tunnel: [1.0 ("Value") -1.0 ("Value")] -> w263
              tunnel: [255.0 ("Value") 1.0 ("Value")] -> w262
              tunnel: [128.0 ("Value") 0.0 ("Value")] -> w261
              tunnel: [64.0 ("Value") 0.5 ("Value")] -> w260
              frame "PWM" {
              }
              frame "Motor", Default {
              }
            }
            n130 = property on="Motor" class="Clust (strict)"("Visible"=TRUE) -> ()  [unwired: 2 in, 2 out]
            n131 = property on="Value" class="Slide (strict)"("Value"=w261, "Scale.Minimum"=w263, "Scale.Maximum"=w262, "Scale.Increment"=w260) -> ()  [unwired: 2 in, 2 out]
            n132 = property on="On/Off" class="Bool (strict)"("Visible"=w265) -> ()  [unwired: 2 in, 2 out]
            n133 = property on="Test Slider" class="Slide (strict)"("Visible"=w265) -> ()  [unwired: 2 in, 2 out]
            n134 = property on="Test Ring" class="Ring (strict)"("Visible"=w265) -> ()  [unwired: 2 in, 2 out]
            n135 = property on="Rev/Fwd" class="Clust (strict)"("Visible"=w265) -> ()  [unwired: 2 in, 2 out]
          }
          frame "Servo" {
            w277 = FALSE ("Visible")
            n136 = call <vilib>:"NT Read Number.vi"("Name"=w279) -> ("Numeric"=w278:dbl)  [unwired: 9 in, 1 out]
            n137 = property on="Test Slider" class="Slide (strict)"("Visible"=TRUE, "Scale.Maximum"=170.0 ("Scale.Range:Maximum")) -> ()  [unwired: 2 in, 2 out]
            n138 = local write "Test Slider"(w278) -> ()
            n139 = property on="Motor" class="Clust (strict)"("Visible"=w277) -> ()  [unwired: 2 in, 2 out]
            n140 = property on="Rev/Fwd" class="Clust (strict)"("Visible"=w277) -> ()  [unwired: 2 in, 2 out]
            n141 = property on="On/Off" class="Bool (strict)"("Visible"=w277) -> ()  [unwired: 2 in, 2 out]
            n142 = property on="Test Ring" class="Ring (strict)"("Visible"=w277) -> ()  [unwired: 2 in, 2 out]
          }
          frame "Relay", "Solenoid" {
            w280 = FALSE ("Visible")
            n143 = property on="Motor" class="Clust (strict)"("Visible"=w280) -> ()  [unwired: 2 in, 2 out]
            n144 = property on="Test Slider" class="Slide (strict)"("Visible"=w280) -> ()  [unwired: 2 in, 2 out]
            n145 = Search and Replace String(input string=w281, search string="/Value  **", replace string="/Direction") -> (result string=w287:string)  [unwired: 5 in, 3 out]
            n146 = property on="Test Ring" class="Ring (strict)"("Visible"=w280) -> ()  [unwired: 2 in, 2 out]
            n147 = call <vilib>:"NT Read String.vi"("Name"=w287) -> ("String"=w285:string)  [unwired: 9 in, 1 out]
            n148 = Equal?(x="Both directions", y=w285) -> (x = y?=w283:bool)
            n149 = Not(x=w283) -> (.not. x?=w284:bool)
            n150 = property on="Rev/Fwd" class="Clust (strict)"("Visible"=w283) -> ()  [unwired: 2 in, 2 out]
            n151 = property on="On/Off" class="Bool (strict)"("Visible"=w284, "Caption.Text"=w282) -> ()  [unwired: 2 in, 2 out]
          }
          frame "Compressor", "Digital Out" {
            w290 = FALSE ("Visible")
            # "Get direction and finish"
            n152 = property on="Motor" class="Clust (strict)"("Visible"=w290) -> ()  [unwired: 2 in, 2 out]
            n153 = property on="Test Slider" class="Slide (strict)"("Visible"=w290) -> ()  [unwired: 2 in, 2 out]
            n154 = property on="Test Ring" class="Ring (strict)"("Visible"=w290) -> ()  [unwired: 2 in, 2 out]
            n155 = property on="On/Off" class="Bool (strict)"("Visible"=TRUE, "Caption.Text"=w291) -> ()  [unwired: 2 in, 2 out]
            n156 = property on="Rev/Fwd" class="Clust (strict)"("Visible"=FALSE) -> ()  [unwired: 2 in, 2 out]
          }
          frame "Camera" {
            n157 = call <vilib>:"Get Last Path Segment.vi"("String in"=w298) -> ("String out"=w299:string)  [unwired: 10 in]
            n158 = property on="On/Off" class="Bool (strict)"("Visible"=FALSE) -> ()  [unwired: 2 in, 2 out]
            n159 = property on="Motor" class="Clust (strict)"("Visible"=FALSE) -> ()  [unwired: 2 in, 2 out]
            n160 = property on="Rev/Fwd" class="Clust (strict)"("Visible"=FALSE) -> ()  [unwired: 2 in, 2 out]
            n161 = case shown="\"White Balance  **\"" w299 {
              tunnel: w298 -> [w305 w314 w323 w332 w341 _ w347]
              tunnel: w297 -> [w303 w311 w320 w329 w338 _ _]
              frame "Size  **" {
                n162 = Index Array(array=w303) -> (element=w302:cluster{string[]})  [unwired: 1 in]
                n163 = call <vilib>:"NT Read String.vi"("Name"=w305) -> ("String"=w304:string)  [unwired: 9 in, 1 out]
                n164 = Unbundle(w302) -> (w300:string[])
                n165 = Match First String(2:w300, 3:w304) -> (0:w301:i32)  [unwired: 1 out]
                n166 = property on="Test Ring" class="Ring (strict)"("Value"=w301, "Strings []"=w300) -> ()  [unwired: 2 in, 2 out]
                n167 = property on="Test Ring" class="Ring (strict)"("Visible"=TRUE) -> ()  [unwired: 2 in, 2 out]
                n168 = property on="Test Slider" class="Slide (strict)"("Visible"=FALSE) -> ()  [unwired: 2 in, 2 out]
              }
              frame "White Balance  **" {
                n169 = Index Array(array=w311, index=1) -> (element=w312:cluster{string[]})
                n170 = call <vilib>:"NT Read String.vi"("Name"=w314) -> ("String"=w313:string)  [unwired: 9 in, 1 out]
                n171 = Unbundle(w312) -> (w309:string[])
                n172 = Match First String(2:w309, 3:w313) -> (0:w308:i32)  [unwired: 1 out]
                n173 = property on="Test Ring" class="Ring (strict)"("Value"=w308, "Strings []"=w309) -> ()  [unwired: 2 in, 2 out]
                n174 = property on="Test Ring" class="Ring (strict)"("Visible"=TRUE) -> ()  [unwired: 2 in, 2 out]
                n175 = property on="Test Slider" class="Slide (strict)"("Visible"=FALSE) -> ()  [unwired: 2 in, 2 out]
              }
              frame "Exposure  **" {
                n176 = Index Array(array=w320, index=2) -> (element=w321:cluster{string[]})
                n177 = call <vilib>:"NT Read String.vi"("Name"=w323) -> ("String"=w322:string)  [unwired: 9 in, 1 out]
                n178 = Unbundle(w321) -> (w317:string[])
                n179 = Match First String(2:w317, 3:w322) -> (0:w318:i32)  [unwired: 1 out]
                n180 = property on="Test Ring" class="Ring (strict)"("Value"=w318, "Strings []"=w317) -> ()  [unwired: 2 in, 2 out]
                n181 = property on="Test Ring" class="Ring (strict)"("Visible"=TRUE) -> ()  [unwired: 2 in, 2 out]
                n182 = property on="Test Slider" class="Slide (strict)"("Visible"=FALSE) -> ()  [unwired: 2 in, 2 out]
              }
              frame "Exposure Priority  **" {
                n183 = Index Array(array=w329, index=3) -> (element=w330:cluster{string[]})
                n184 = call <vilib>:"NT Read String.vi"("Name"=w332) -> ("String"=w331:string)  [unwired: 9 in, 1 out]
                n185 = Unbundle(w330) -> (w326:string[])
                n186 = Match First String(2:w326, 3:w331) -> (0:w327:i32)  [unwired: 1 out]
                n187 = property on="Test Ring" class="Ring (strict)"("Value"=w327, "Strings []"=w326) -> ()  [unwired: 2 in, 2 out]
                n188 = property on="Test Ring" class="Ring (strict)"("Visible"=TRUE) -> ()  [unwired: 2 in, 2 out]
                n189 = property on="Test Slider" class="Slide (strict)"("Visible"=FALSE) -> ()  [unwired: 2 in, 2 out]
              }
              frame "Color Enable  **" {
                n190 = Index Array(array=w338, index=4) -> (element=w339:cluster{string[]})
                n191 = call <vilib>:"NT Read String.vi"("Name"=w341) -> ("String"=w340:string)  [unwired: 9 in, 1 out]
                n192 = Unbundle(w339) -> (w335:string[])
                n193 = Match First String(2:w335, 3:w340) -> (0:w336:i32)  [unwired: 1 out]
                n194 = property on="Test Ring" class="Ring (strict)"("Value"=w336, "Strings []"=w335) -> ()  [unwired: 2 in, 2 out]
                n195 = property on="Test Ring" class="Ring (strict)"("Visible"=TRUE) -> ()  [unwired: 2 in, 2 out]
                n196 = property on="Test Slider" class="Slide (strict)"("Visible"=FALSE) -> ()  [unwired: 2 in, 2 out]
              }
              frame Default {
                n197 = property on="Test Ring" class="Ring (strict)"("Visible"=FALSE) -> ()  [unwired: 2 in, 2 out]
                n198 = property on="Test Slider" class="Slide (strict)"("Visible"=FALSE) -> ()  [unwired: 2 in, 2 out]
              }
              frame "Brightness  **", "Color Level  **", "Compression  **", "FPS  **", "Sharpness  **" {
                n199 = call <vilib>:"NT Read Number.vi"("Name"=w347) -> ("Numeric"=w346:dbl)  [unwired: 9 in, 1 out]
                n200 = local write "Test Slider"(w346) -> ()
                n201 = property on="Test Slider" class="Slide (strict)"("Visible"=TRUE, "Scale.Maximum"=100.0 ("Scale.Range:Maximum")) -> ()  [unwired: 2 in, 2 out]
                n202 = property on="Test Ring" class="Ring (strict)"("Visible"=FALSE) -> ()  [unwired: 2 in, 2 out]
              }
            }
          }
        }
        n203 = property on="Progress" class="Clust (strict)"("Visible"=FALSE) -> ()  [unwired: 2 in, 2 out]
      }
      event "Test Name": Mouse Enter {
        # "Populate the ring with the list of tests"
        n204 = event-data() -> ()  [unwired: 1 in, 1 out]
        n205 = call <vilib>:"NT Read String Array.vi"("Name"="TestMode/TestList") -> ("String Array"=w355:string[])  [unwired: 9 in, 1 out]
        n206 = Build Array (concatenate)("Select the test to run...", w355) -> (w354:string[])
        n207 = property on="Test Name" class="Ring (strict)"("Strings []"=w354) -> ()  [unwired: 2 in, 2 out]
      }
      event "Test Name": Value Change {
        w357 = FALSE ("Visible")
        # "Tell the robot the test name to run"
        n208 = event-data() -> ("NewVal"=w361:u16)  [unwired: 1 in]
        n209 = property on="Test Name" class="Ring (strict)"() -> ("Strings []"=w362:string[])  [unwired: 2 in, 2 out]
        n210 = local write "Progress"(T14 {"Test Progress"=0, "Test Progress Text"=""} ("Progress")) -> ()
        n211 = Index Array(array=w362, index=w361) -> (element=w360:string)
        n212 = call <vilib>:"NT Write String.vi"("String"=w360, "Name"="TestMode/TestName") -> ()  [unwired: 9 in, 1 out]
        n213 = property on="Progress" class="Clust (strict)"("Visible"=TRUE) -> ()  [unwired: 2 in, 2 out]
        n214 = property on="Motor" class="Clust (strict)"("Visible"=w357) -> ()  [unwired: 2 in, 2 out]
        n215 = property on="Test Slider" class="Slide (strict)"("Visible"=w357) -> ()  [unwired: 2 in, 2 out]
        n216 = property on="On/Off" class="Bool (strict)"("Visible"=w357) -> ()  [unwired: 2 in, 2 out]
        n217 = property on="Rev/Fwd" class="Clust (strict)"("Visible"=w357) -> ()  [unwired: 2 in, 2 out]
        n218 = property on="Test Ring" class="Ring (strict)"("Visible"=w357) -> ()  [unwired: 2 in, 2 out]
      }
      event "Listbox": Double Click {
        # "Shift clears all"
        # "Update symbols on the listbox"
        n219 = event-data() -> ("PlatMods.Shift"=w365:bool, "Row"=w367:i32)  [unwired: 1 in]
        n220 = case shown="True" w365 {
          tunnel: w367 -> [w371 _]
          tunnel: 1 -> [w370 _]
          frame False {
            n221 = property on="Listbox" class="LstBox (strict)"() -> ("Item Symbols"=w369:i32[])  [unwired: 2 in, 2 out]
            n222 = Replace Array Subset(array=w369, new element=w370, index=w371) -> (w368:i32[])
            n223 = property on="Listbox" class="LstBox (strict)"("Item Symbols"=w368) -> ()  [unwired: 2 in, 2 out]
          }
          frame True {
            w372 = 0 ("Top Row")
            n224 = property on="Listbox" class="LstBox (strict)"() -> ("Number of Rows"=w374:u32)  [unwired: 2 in, 2 out]
            n225 = Initialize Array(0, w374) -> (w373:i32[])
            n226 = property on="Listbox" class="LstBox (strict)"("Top Row"=w372, "Value"=w372, "Item Symbols"=w373) -> ()  [unwired: 2 in, 2 out]
          }
        }
      }
      event "Listbox": Key Down {
        # "Update symbols on the listbox\nLeft and right keys check and uncheck"
        n227 = event-data() -> ("VKey"=w378:T33)  [unwired: 1 in]
        n228 = case shown="\"Left\", \"Right\"" w378 {
          selector: w378 -> [w383 _]
          tunnel: eventvkey."Left" ("VKey") -> [w381 _]
          frame "Left", "Right" {
            n229 = Equal?(x=w381, y=w383) -> (x = y?=w382:bool)
            n230 = Select(t=0, s=w382, f=1) -> (s? t:f=w384:i32)
            n231 = property on="Listbox" class="LstBox (strict)"() -> ("Item Symbols"=w387:i32[])  [unwired: 2 in, 2 out]
            n232 = Replace Array Subset(array=w387, new element=w384, index="Listbox") -> (w386:i32[])
            n233 = property on="Listbox" class="LstBox (strict)"("Item Symbols"=w386) -> ()  [unwired: 2 in, 2 out]
          }
          frame Default {
          }
        }
      }
      event "DB Camera Config": Value Change {
        # "Show or hide the cluster of controls, store in ini file"
        n234 = event-data() -> ("NewVal"=w391:bool)  [unwired: 1 in]
        n235 = case shown="False" w391 {
          tunnel: w390 -> [w400 _]
          tunnel: [w393 w411] -> w389
          tunnel: w388 -> [w392 w411]
          frame False {
            w407 = "Camera"
            w410 = FALSE ("Visible")
            n236 = local read "Camera Settings"() -> (w399:T4)
            n237 = Index Array(array=w400) -> (element=w403:cluster{string[]})  [unwired: 1 in]
            n238 = Unbundle(w399) -> ("Frame Rate"=w398:i32, "Compression"=w397:i32, "Size"=w401:u16)
            n239 = Unbundle(w403) -> (w402:string[])
            n240 = Index Array(array=w402, index=w401) -> (element=w396:string)
            n241 = call-poly <vilib>:"Write Key.vi"("section"=w407, "value"=w396, "key"="Size", "refnum"=w392) -> ("refnum out"=w409:T31)  [unwired: 2 in, 5 out]
            n242 = call-poly <vilib>:"Write Key.vi"("section"=w407, "value"=w398, "key"="FrameRate", "refnum"=w409) -> ("refnum out"=w408:T31)  [unwired: 1 in, 6 out]
            n243 = property on="Camera Settings" class="Clust (strict)"("Visible"=w410) -> ()  [unwired: 2 in, 2 out]
            n244 = local write "DB Camera Config"(w410) -> ()
            n245 = call-poly <vilib>:"Write Key.vi"("section"=w407, "value"=w397, "key"="Compression", "refnum"=w408) -> ("refnum out"=w394:T31)  [unwired: 1 in, 6 out]
            n246 = call <vilib>:"Close Config Data.vi"("refnum"=w394) -> ("file path"=w395:path)  [unwired: 2 in, 8 out]
            n247 = call <vilib>:"Open Config Data.vi"("configuration file path"=w395) -> ("refnum"=w393:T31)  [unwired: 8 in, 2 out]
          }
          frame True {
            n248 = property on="Camera Settings" class="Clust (strict)"("Visible"=TRUE) -> ()  [unwired: 2 in, 2 out]
          }
        }
      }
      event "Camera Settings": Value Change {
        # "Update summary string when any elements of DB camera change"
        n249 = event-data() -> ("NewVal"=w424:T4)  [unwired: 1 in]
        n250 = Index Array(array=w420) -> (element=w419:cluster{string[]})  [unwired: 1 in]
        n251 = Unbundle(w424) -> ("Frame Rate"=w415:i32, "Compression"=w414:i32, "Size"=w417:u16)
        n252 = Unbundle(w419) -> (w418:string[])
        n253 = Index Array(array=w418, index=w417) -> (element=w416:string)
        n254 = Format Into String(format string="%s   %dfps   %d%%", w416, w415, w414) -> (resulting string=w421:string)  [unwired: 2 in, 1 out]
        n255 = Build Array(w421) -> (w422:string[])
        n256 = property on="DB Camera Config" class="Bool (strict)"("Strings [4]"=w422) -> ()  [unwired: 2 in, 2 out]
      }
      event "Motor.Enable": Value Change {
        # "When the test mode otor enable helper is set, update that\ntree row item's value"
        n257 = event-data() -> ("NewVal"=w430:bool)  [unwired: 1 in]
        n258 = Unbundle("Motor") -> ("Value"=w429:dbl)  [unwired: 1 out]
        n259 = Select(t=w429, s=w430, f=0.0) -> (s? t:f=w427:dbl)
        n260 = call <vilib>:"NT Write Number.vi"("Numeric"=w427, "Name"=w426) -> ()  [unwired: 9 in, 1 out]
      }
      event "Test Slider": Value Change {
        # "When the test mode slider helper is set, update that\ntree row item's value"
        n261 = event-data() -> ("NewVal"=w433:dbl)  [unwired: 1 in]
        n262 = call <vilib>:"NT Write Number.vi"("Numeric"=w433, "Name"=w434) -> ()  [unwired: 9 in, 1 out]
      }
      event "On/Off": Value Change {
        # "When the test mode on/off helper value is set, update that\ntree row item's value"
        n263 = event-data() -> ("NewVal"=w438:bool)  [unwired: 1 in]
        n264 = Boolean To (0,1)(Boolean=w438) -> (0, 1=w437:i16)
        n265 = call <vilib>:"NT Write Number.vi"("Numeric"=w437, "Name"=w436) -> ()  [unwired: 9 in, 1 out]
      }
      event "Rev/Fwd": Value Change {
        # "When the test mode helper value for relays is set, update that\ntree row item's value"
        n266 = event-data() -> ("NewVal.Forward"=w446:bool, "NewVal.Reverse"=w445:bool)  [unwired: 1 in]
        n267 = Boolean To (0,1)(Boolean=w446) -> (0, 1=w442:i16)
        n268 = Boolean To (0,1)(Boolean=w445) -> (0, 1=w444:i16)
        n269 = Negate(x=w444) -> (-x=w443:i16)
        n270 = Add(x=w442, y=w443) -> (x+y=w441:i16)
        n271 = call <vilib>:"NT Write Number.vi"("Numeric"=w441, "Name"=w440) -> ()  [unwired: 9 in, 1 out]
      }
      event "Test Ring": Value Change {
        # "When a test mode helper value is selected from the ring,\nset the tree item's variable to the string value"
        n272 = event-data() -> ("NewVal"=w450:u16)  [unwired: 1 in]
        n273 = property on="Test Ring" class="Ring (strict)"() -> ("Strings []"=w451:string[])  [unwired: 2 in, 2 out]
        n274 = Index Array(array=w451, index=w450) -> (element=w449:string)
        n275 = call <vilib>:"NT Write String.vi"("String"=w449, "Name"=w448) -> ()  [unwired: 9 in, 1 out]
      }
      event "Rec Mode": Value Change {
        # "Update globals for recording mode and path to read log from.\nClear when logging and let NetworkTables set path for vision to\nuse."
        n276 = event-data() -> ("NewVal"=w461:enum32{"Stop", "Record", "Playback"})  [unwired: 1 in]
        n277 = global write "WPI_DashboardLogging Global.vi" "Logging Filename"(path "") -> ()
        n278 = case shown="\"Playback\"" w461 {
          tunnel: w460 -> [_ w463 w471]
          tunnel: [_ _ w470] -> w457
          tunnel: [_ _ w469] -> _
          tunnel: w455 -> [_ _ w467]
          tunnel: cluster{i32, i32} {-250, 170} -> [_ _ w466]
          tunnel: [_ _ T34 {"Image Size"=TRUE, "Image Type"=TRUE, "Pixel Value"=TRUE, "ROI Information"=TRUE, "Zoom Factor"=FALSE} ("Image Information Shown:All Elements")] -> w453
          tunnel: [_ _ TRUE ("Zoom Factor")] -> w452
          frame Default {
          }
          frame "Stop", "Record" {
            # "Place Window too"
            n279 = invoke class="VI" method="FP.Close"(reference=w463) -> (reference out=w462:refnum<vi>)  [unwired: 2 in, 2 out]
            n280 = invoke class="VI" method="Abort VI"(reference=w462) -> ()  [unwired: 2 in, 3 out]
          }
          frame "Playback" {
            n281 = call "Open Playback Panel.vi"("Offset"=w466, "DB VI Ref"=w467, "Playback in"=w471) -> ("Playback out"=w468:refnum<vi>)  [unwired: 8 in]
            n282 = register-events(w468) -> (reference out=w470:refnum<event-registration>, error out=w469:errorcluster)  [unwired: 2 in]
          }
        }
        n283 = global write "WPI_DashboardLogging Global.vi" "Recording"(w461) -> ()
        n284 = property on="Camera Image" class="ImageControl"("Image Information Shown"=w453, "Image Information Visible"=w452) -> ()  [unwired: 2 in, 2 out]
        n285 = call <vilib>:"WPI_DashboardNT Log FieldName Cache.vi"("Operation"=enum16{"Lookup/Add", "Index", "Clear"}."Clear") -> ()  [unwired: 8 in, 3 out]
      }
      event Panel Close {
        w472 = enum32{"Stop", "Record", "Playback"}."Stop" ("Rec Mode")
        # "Playback window has been closed, abort"
        n286 = event-data() -> ()  [unwired: 1 in, 4 out]
        n287 = local write "Rec Mode"(w472) -> ()
        n288 = global write "WPI_DashboardLogging Global.vi" "Recording"(w472) -> ()
      }
      event Panel Close {
        # "Abort playback window and ourself"
        n289 = event-data() -> ()  [unwired: 1 in, 4 out]
        n290 = invoke class="VI" method="FP.Close"(reference=w477) -> (reference out=w476:refnum<vi>)  [unwired: 2 in, 2 out]
        n291 = invoke class="VI" method="Abort VI"(reference=w476) -> (error out=w475:errorcluster)  [unwired: 2 in, 2 out]
        n292 = invoke class="VI" method="Abort VI"(error in=w475) -> ()  [unwired: 2 in, 3 out]
      }
      event "Vision": Value Change {
        # "Enable/Disable Compression slider.\nHW USB is hard-coded into the camera"
        n293 = event-data() -> ("NewVal"=w483:u16)  [unwired: 1 in]
        n294 = Equal?(x=w483, y=u32 2 ("milliseconds to wait")) -> (x = y?=w481:bool)
        n295 = Select(t=T35."Disabled and Grayed Out" ("Disabled"), s=w481, f=T35."Enabled" ("Disabled")) -> (s? t:f=w478:T35)
        n296 = property on="Compression" class="Slide (strict)"("DisabledEnum"=w478) -> ()  [unwired: 2 in, 2 out]
      }
    }
  }
  n297 = while {
    tunnel: w44 -> [w486]
    i -> [w489]
    stop <- FALSE stop-if-true
    n298 = Wait (ms)(milliseconds to wait=u32 100) -> ()  [unwired: 1 out]
    n299 = case shown="\"Playback\"" "Rec Mode" {
      tunnel: w489 -> [_ _ w504]
      tunnel: [u32 2829099 ("Base Color") u32 11141120 ("Target Color") w493] -> w485
      frame "Stop", Default {
        # "Reset the color, extra updates don't cost much"
      }
      frame "Record" {
      }
      frame "Playback" {
        # "Playback"
        n300 = Quotient & Remainder(x=w504, y=u32 50 ("milliseconds to wait")) -> (x-y*floor(x/y)=w500:u32)  [unwired: 1 out]
        n301 = Divide(x=w500, y=u32 50 ("milliseconds to wait")) -> (x/y=w497:dbl)
        n302 = Multiply(x=6.283185307179586, y=w497) -> (x*y=w502:dbl)
        n303 = Sine(x=w502) -> (sin(x)=w501:dbl)
        n304 = Absolute Value(x=w501) -> (abs(x)=w494:dbl)
        n305 = call "Interpolate RGB Color.vi"("Proportion"=w494, "Target Color"=u32 30976, "Base Color"=u32 2829099) -> ("Result Color"=w493:u32)  [unwired: 8 in]
      }
    }
    n306 = property class="Pane"(reference=w486, "PaneColor"=w485) -> ()  [unwired: 1 in, 2 out]
  }
  n307 = TCP Create Listener(10:u16 1741 ("timeout ms (25000)")) -> (3:w7:refnum<k5>)  [unwired: 4 in, 2 out]
  n308 = while {
    tunnel: w7 -> [w506]
    stop <- FALSE stop-if-true
    n309 = TCP Wait On Listener(11:w506) -> (4:w505:refnum<k5>)  [unwired: 3 in, 4 out]
    n310 = local write "TCP"(w505) -> ()
  }
  n311 = property on="On/Off" class="Bool (strict)"("Visible"=w12) -> ()  [unwired: 2 in, 2 out]
  n312 = property on="Motor" class="Clust (strict)"("Visible"=w12) -> ()  [unwired: 2 in, 2 out]
  n313 = property on="Progress" class="Clust (strict)"("Visible"=w12) -> ()  [unwired: 2 in, 2 out]
  n314 = property on="Test Ring" class="Ring (strict)"("Visible"=w12) -> ()  [unwired: 2 in, 2 out]
  n315 = property on="Rev/Fwd" class="Clust (strict)"("Visible"=w12) -> ()  [unwired: 2 in, 2 out]
  n316 = property on="Camera Settings" class="Clust (strict)"("Visible"=w12) -> ()  [unwired: 2 in, 2 out]
  n317 = local write "DB Camera Config"(w12) -> ()
  n318 = global write "WPI_DashboardLogging Global.vi" "Recording"(w38) -> ()
  n319 = local write "Rec Mode"(w38) -> ()
  n320 = Current VI's Path() -> (path=w6:path)
  n321 = Strip Path(path=w6) -> (stripped path=w5:path)  [unwired: 1 out]
  n322 = while {
    tunnel: w5 -> [w511]
    stop <- FALSE stop-if-true
    n323 = Wait (ms)(milliseconds to wait=u32 3000) -> ()  [unwired: 1 out]
    n324 = Path Type(1:"Folder Location") -> (0:w512:i16)
    n325 = case shown="1" w512 {
      tunnel: "Folder Location" -> [w516 w519]
      tunnel: [w516 w517] -> w510
      tunnel: w511 -> [_ w518]
      frame 0, Default {
      }
      frame 1 {
        n326 = Build Path(base path=w518, name or relative path=w519) -> (appended path=w517:path)
      }
    }
    n327 = for {
      tunnel: [w522] -> w509 mode=concatenating
      tunnel: w510 -> [w521]
      tunnel: string[] ["*.jpg", "*.png", "*.bmp"] -> [w520] mode=indexing
      n328 = List Folder(path=w521, pattern=w520) -> (filenames=w522:string[])  [unwired: 2 in, 3 out]
    }
    n329 = local write "Image Path"(w510) -> ()
    n330 = local write "image files"(w509) -> ()
    n331 = property on="Images" class="LstBox (strict)"("Item Names"=w509) -> ()  [unwired: 2 in, 2 out]
  }
